vi "Set Extension.vi"(8 "error in (no error)":errorcluster, 11 "TDMS Report":refnum<class "Wind TDMS Report.lvclass">) -> (0 "error out":errorcluster, 3 "TDMS Report out":refnum<class "Wind TDMS Report.lvclass">)   [LabVIEW 2009, in "Wind TDMS Report.lvclass"]
doc: "This dynamic dispatch VI overrides the parent and sets the unique file extension for the child class.\n\nAAL 9/09"
uses:
  Wind TDMS Report.lvclass
  Wind Report/Wind Report.lvclass
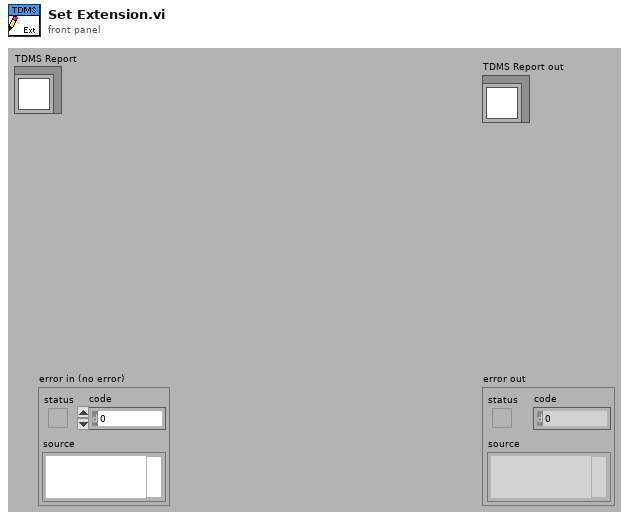
[diagram p1: front panel]
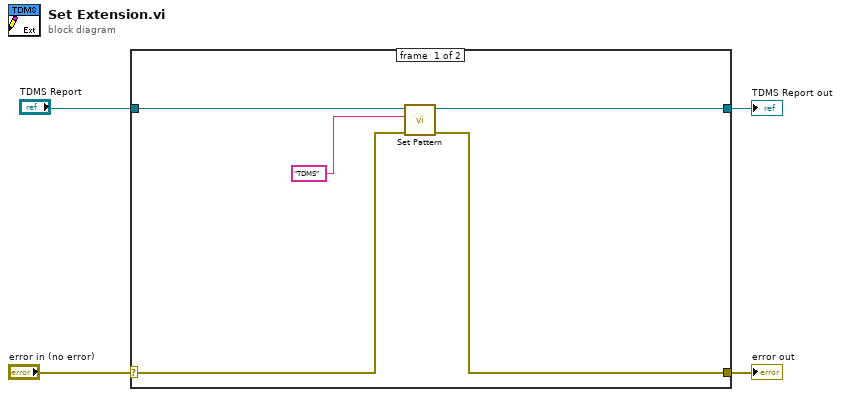
[diagram p0: block diagram]
diagram:
  n1 = case shown="No Error" "error in (no error)" {
    selector: "error in (no error)" -> [w8 w11]
    tunnel: [w7 w11] -> w3
    tunnel: [w9 w10] -> w2
    tunnel: "TDMS Report" -> [w6 w10]
    frame #0 {
      n2 = call "Set Pattern.vi"("error in (no error)"=w8, "Pattern"="TDMS", "Report.lvclass in"=w6) -> ("error out"=w7:errorcluster, "Report.lvclass out"=w9:refnum<class "Wind TDMS Report.lvclass">)  [unwired: 7 in]
    }
    frame #1 {
    }
  }
  "error out" <- w3
  "TDMS Report out" <- w2
